vi "Tags.vi"() -> ()   [LabVIEW 2011]
panel:
  in  "Abort Recipe":bool
  in  "Stop":bool
  out "Waste ON":bool
  out "Intake ON":bool
  out "Agitation ON":bool
  out "pH Override":bool
  in  "pH Override SP":dbl
  in  "pH Recipe SP":dbl
  out "Temp Override":bool
  in  "Temp Override SP":dbl
  in  "Temp Recipe SP":dbl
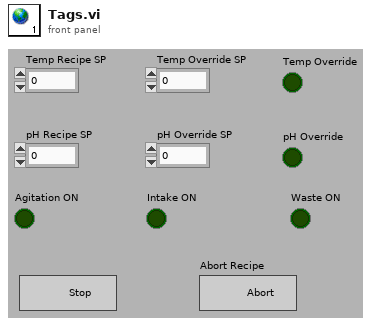
[diagram p1: front panel]
diagram:
